vi "A-Lockin_Vsg.vi"(7 "Remote Lockin Address":string, 8 "error in (no error)":errorcluster, 11 "SweepControl.lvclass":refnum<class "SweepControl.lvclass">) -> (0 "error out":errorcluster)   [LabVIEW 2016, in "Transport.lvclass"]
uses:
  Transport.lvclass
  <userlib>/LevyLab/Lockin-Multichannel/Typedefs/AO-cluster.ctl
  <userlib>/LevyLab/Lockin-Multichannel/Typedefs/AO_Amp-array.ctl
  <userlib>/LevyLab/Lockin-Multichannel/Typedefs/AO_DC-array.ctl
  <userlib>/LevyLab/Lockin-Multichannel/Typedefs/AO_f-array.ctl
  <userlib>/LevyLab/Lockin-Multichannel/Typedefs/AO_phi-array.ctl
  <userlib>/LevyLab/Lockin-Multichannel/Typedefs/Function-array.ctl
  <userlib>/LevyLab/Lockin-Multichannel/Typedefs/Function-enum.ctl
  SweepControl/SweepControl.lvclass
  <userlib>/LevyLab/Levylab Instruments/Instrument Types/Cryostat/Instrument.Cryostat.lvclass
  <userlib>/LevyLab/LV to ITX/LVtoITX.lvclass
  Control Experiment/Control Experiment.lvclass
panel:
  in  "Tab Control":enum32{"lockin/SG Control", "Data", "Other"}(tab)
  out "elapsed time (s)":u32=76
  in  "Side Gate Channel(s)":i32[](array[numeric])
  in  "Channels: AO":T1={"AO amp (V)"=[0.0, 0.0, 0.0, 0.0, 0.0, 0.0, 0.0, 0.0], "AO DC (V)"=[0.0, 0.0, 0.0, 0.0, 0.0, 0.0, 0.0, 0.0], "AO f (Hz)"=[13.0, 13.0, 13.0, 13.0, 13.0, 13.0, 13.0, 13.0], "AO phi (°)"=[0.0, 0.0, 0.0, 0.0, 0.0, 0.0, 0.0, 0.0], "function"=[enum."Sine", enum."Sine", enum."Sine", enum."Sine", enum."Sine", enum."Sine", enum."Sine", enum."Sine"], "I+"=[]} {"AO f (Hz)" min=0.001 max=10000.0; "AO DC (V)" format="%.3p"; "AO amp (V)" format="%.3p"}
  in  "Vmax (end)":dbl=0.7 format="%#_3p"
  in  "Vmin (start)":dbl=-0.15 format="%#_3p"
  in  "dV":dbl=0.0005 format="%#_3p"
  in  "Experiment Comments":string="describe only the experiment you're doing right now"
  in  "Experiment folder":string="Experiment folder"
  out "T (mK)":dbl
  in  "wait after setting Vsg (ms)":u32
  in  "Initial wait (ms)":u32=10000
  in  "Physical Channel":tag="Dev2/ao0" caption="Back Gate Channel"
  in  "Sweep":enum16{"Vsg", "Vbg"}(ring)
  in  "cycles (1,2,...)":i32=1 min=1 step=1
  in  "phase":dbl
  out "ramp rate":dbl=0.2 format="%#_13g"
  out "Field (T)":dbl=0.5 format="%#_13g"
  in  "function (ramp)":enum16{"Ramp", "Triangle", "Sine"}(ring)
  in  "set \"Vsg\" to initial value?":bool
  out "time b/w points (ms)":u32=76
  in  "stop":bool
  out "X Lockins":cluster{"Y":dbl[], "Y":dbl[]}[](graph)
  in  "V1":i32=1 min=1
  in  "Current":i32=1 min=1
  in  "V2":i32=1 min=1
  out "X Lockins 2":cluster{"Y":dbl[], "Y":dbl[]}[](graph)
  out "G4T":cluster{"Y":dbl[], "Y":dbl[]}[](graph)
  # "1"
  # "2"
  # "3"
  # "4"
  # "5"
  # "6"
  # "7"
  # "8"
  # "If V1 /= V2:\nR = (V1-V2)/I\nIf V1 = V2:\nR = V1/I"
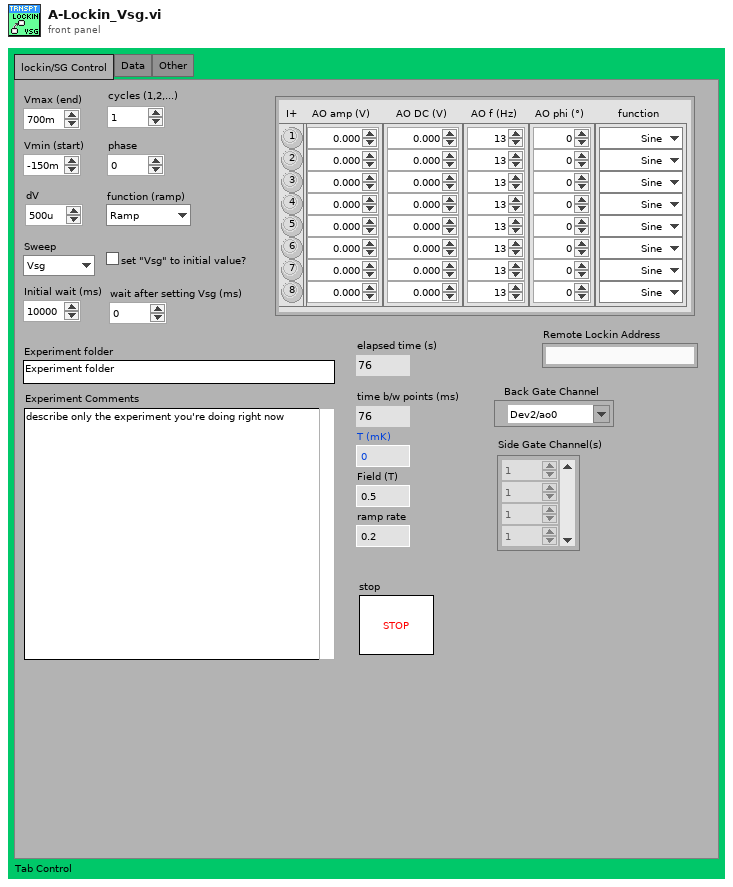
[diagram p1: front panel]
types:
  T1 = typedef "AO-cluster.ctl" = cluster{"AO amp (V)":T2, "AO DC (V)":T3, "AO f (Hz)":T4, "AO phi (°)":T5, "function":T6, "I+":bool[]}
  T2 = typedef "AO_Amp-array.ctl" = dbl[]
  T3 = typedef "AO_DC-array.ctl" = dbl[]
  T4 = typedef "AO_f-array.ctl" = dbl[]
  T5 = typedef "AO_phi-array.ctl" = dbl[]
  T6 = typedef "Function-array.ctl" = T7[]
  T7 = typedef "Function-enum.ctl" = enum16{"Sine", "Triangle", "Square", "Sawtooth"}
  T8 = cluster{"Temperature":refnum<class "Instrument.Cryostat.lvclass">, "Magnet":refnum<class "Instrument.Cryostat.lvclass">, "Rotator":refnum<class "Instrument.Cryostat.lvclass">, "Level":refnum<class "Instrument.Cryostat.lvclass">}
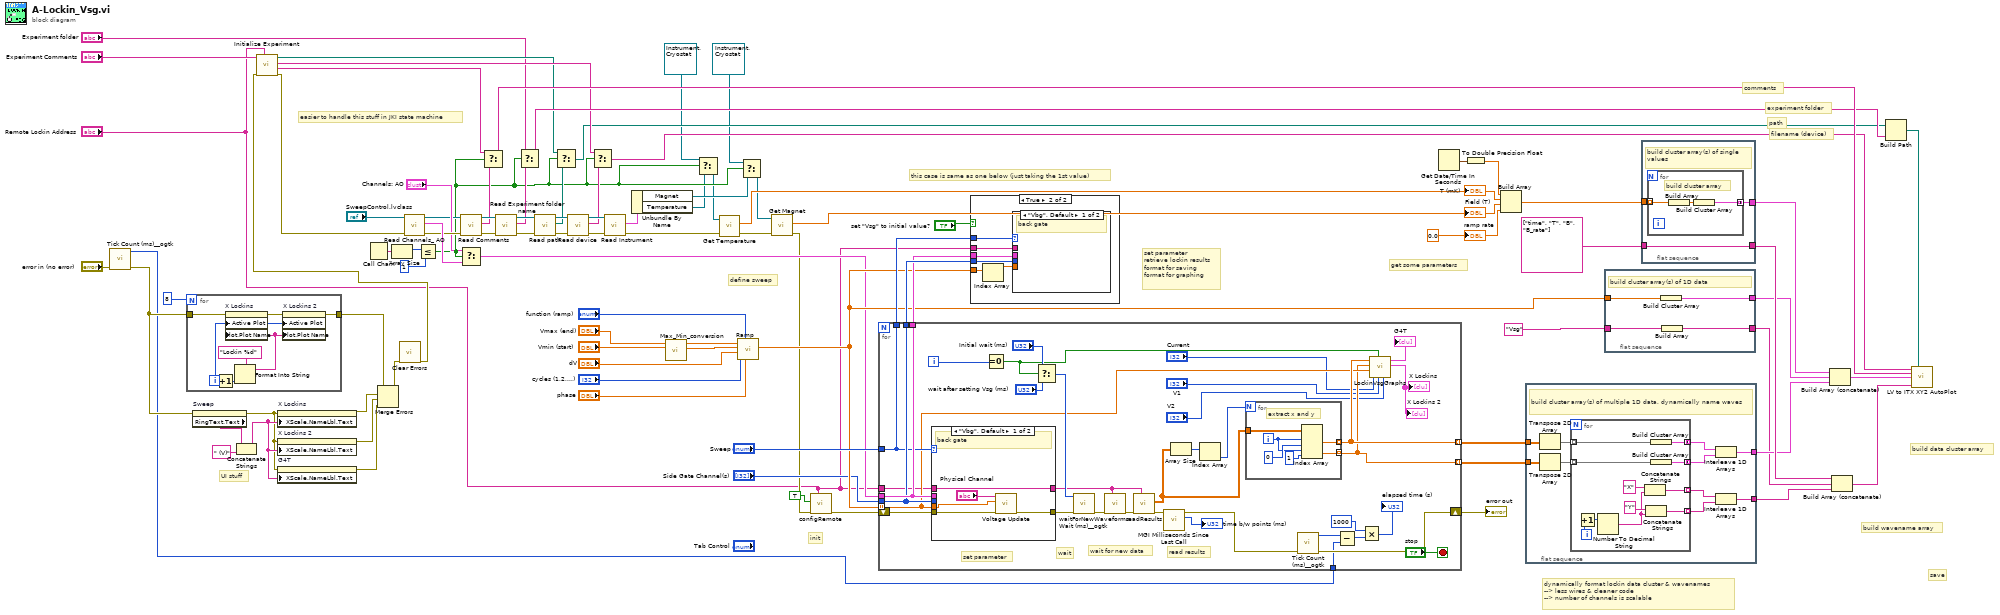
[diagram p0: block diagram]
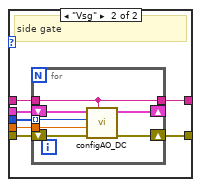
[diagram p2: hidden frame]
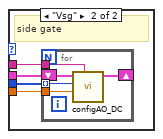
[diagram p4: hidden frame]
diagram:
  w69 = 0.0
  # "UI stuff"
  # "easier to handle this stuff in JKI state machine"
  # "filename (device)"
  # "path"
  # "comments"
  # "experiment folder"
  # "define sweep"
  # "get some parameters"
  # "set parameter\nretrieve lockin results\nformat for saving\nformat for graphing"
  # "save"
  # "this case is same as one below (just taking the 1st value)"
  # "init"
  # "build data cluster array"
  # "build wavename array"
  # "dynamically format lockin data cluster & wavenames\n--> less wires & cleaner code\n--> number of channels is scalable"
  n1 = call <userlib>:"Tick Count (ms)__ogtk.vi"("error in (no error)"="error in (no error)") -> ("error out"=w16:errorcluster, "millisecond timer value"=w4:u32)  [unwired: 9 in]
  n2 = for {
    N: 8 -> [_]
    tunnel: [w95] -> w10
    tunnel: w16 -> [w100]
    i -> [w98]
    n3 = Increment(x=w98) -> (x+1=w96:i32)
    n4 = Format Into String(format string="Lockin %d", w96) -> (resulting string=w99:string)  [unwired: 2 in, 1 out]
    n5 = property on="X Lockins" class="XYGraph (strict)"(error in=w100, "Active Plot"=w98, "Plot.Plot Name"=w99) -> (error out=w97:errorcluster)  [unwired: 1 in, 1 out]
    n6 = property on="X Lockins 2" class="XYGraph (strict)"(error in=w97, "Active Plot"=w98, "Plot.Plot Name"=w99) -> (error out=w95:errorcluster)  [unwired: 1 in, 1 out]
  }
  n7 = property on="Sweep" class="Enum (strict)"(error in=w16) -> (error out=w11:errorcluster, "RingText.Text"=w13:string)  [unwired: 1 in, 1 out]
  n8 = Concatenate Strings(w13, " (V)" ("string")) -> (w12:string)
  n9 = property on="X Lockins" class="XYGraph (strict)"(error in=w11, "XScale.NameLbl.Text"=w12) -> (error out=w9:errorcluster)  [unwired: 1 in, 1 out]
  n10 = property on="X Lockins 2" class="XYGraph (strict)"(error in=w11, "XScale.NameLbl.Text"=w12) -> (error out=w8:errorcluster)  [unwired: 1 in, 1 out]
  n11 = property on="G4T" class="XYGraph (strict)"(error in=w11, "XScale.NameLbl.Text"=w12) -> (error out=w7:errorcluster)  [unwired: 1 in, 1 out]
  n12 = Call Chain() -> (call chain=w64:string[])
  n13 = Merge Errors(w10, w9, w8, w7) -> (w6:errorcluster)
  n14 = Array Size(array=w64) -> (size(s)=w63:i32)
  n15 = call <vilib>:"Clear Errors.vi"("error in (no error)"=w6) -> ("error out"=w5:errorcluster)  [unwired: 5 in, 1 out]
  n16 = call "Initialize Experiment.vi"("lockin address"="Remote Lockin Address", "error in (no error)"=w5, "Experiment Comments"="Experiment Comments") -> ("error out"=w31:errorcluster, "Comments"=w32:string, "device"=w38:string, "path"=w36:path)  [unwired: 5 in]
  n17 = call-dynamic "Read Channels_ AO.vi"("error in (no error)"=w31, "SweepControl in"="SweepControl.lvclass") -> ("error out"=w56:errorcluster, "Channels: AO"=w61:T1, "SweepControl out"=w54:refnum<class "SweepControl.lvclass">)  [unwired: 7 in]
  n18 = Less Or Equal?(x=w63, y=1) -> (x <= y?=w23:bool)
  n19 = call-dynamic "Read Comments.vi"("error in (no error)"=w56, "SweepControl in"=w54) -> ("error out"=w58:errorcluster, "Comments"=w49:string, "SweepControl out"=w57:refnum<class "SweepControl.lvclass">)  [unwired: 7 in]
  n20 = Select(t="Channels: AO", s=w23, f=w61) -> (s? t:f=w59:T1)
  n21 = Select(t=w32, s=w23, f=w49) -> (s? t:f=w47:string)
  n22 = call-dynamic "Read Experiment folder name.vi"("error in (no error)"=w58, "SweepControl in"=w57) -> ("error out"=w53:errorcluster, "Experiment folder name"=w48:string, "SweepControl out"=w50:refnum<class "SweepControl.lvclass">)  [unwired: 7 in]
  n23 = Select(t="Experiment folder", s=w23, f=w48) -> (s? t:f=w41:string)
  n24 = call-dynamic "Read path.vi"("error in (no error)"=w53, "SweepControl in"=w50) -> ("error out"=w52:errorcluster, "path"=w40:path, "SweepControl out"=w51:refnum<class "SweepControl.lvclass">)  [unwired: 7 in]
  n25 = Select(t=w36, s=w23, f=w40) -> (s? t:f=w35:path)
  n26 = call-dynamic "Read device.vi"("error in (no error)"=w52, "SweepControl in"=w51) -> ("error out"=w45:errorcluster, "device"=w39:string, "SweepControl out"=w46:refnum<class "SweepControl.lvclass">)  [unwired: 7 in]
  n27 = Select(t=w38, s=w23, f=w39) -> (s? t:f=w37:string)
  n28 = call-dynamic "Read Instrument.vi"("error in (no error)"=w45, "SweepControl in"=w46) -> ("error out"=w28:errorcluster, "Instrument"=w24:T8)  [unwired: 7 in, 1 out]
  n29 = Unbundle By Name(w24) -> ("Magnet"=w22:refnum<class "Instrument.Cryostat.lvclass">, "Temperature"=w21:refnum<class "Instrument.Cryostat.lvclass">)
  n30 = call <userlib>:"Max_Min_conversion.vi"("Min"="Vmin (start)", "Max"="Vmax (end)") -> ("offset"=w91:dbl, "Amplitude"=w92:dbl)  [unwired: 8 in]
  n31 = Select(t=refnum<class "Instrument.Cryostat.lvclass"> refnum ("Magnet"), s=w23, f=w21) -> (s? t:f=w20:refnum<class "Instrument.Cryostat.lvclass">)
  n32 = call-dynamic "Get Temperature.vi"("error in (no error)"=w28, "Instrument.Cryostat in"=w20) -> ("error out"=w29:errorcluster, "Temperature (K)"=w25:dbl)  [unwired: 6 in, 2 out]
  "T (mK)" <- w25
  n33 = call <userlib>:"Ramp.vi"("phase"="phase", "function (ramp)"="function (ramp)", "cycles (1,2,...)"="cycles (1,2,...)", "step size"="dV", "offset"=w91, "amplitude"=w92) -> ("Waveform Graph"=w66:dbl[])  [unwired: 3 in, 2 out]
  n34 = Select(t=refnum<class "Instrument.Cryostat.lvclass"> refnum ("Magnet"), s=w23, f=w22) -> (s? t:f=w19:refnum<class "Instrument.Cryostat.lvclass">)
  n35 = call-dynamic "Get Magnet.vi"("error in (no error)"=w29, "Instrument.Cryostat in"=w19) -> ("error out"=w27:errorcluster, "B Field (T)"=w26:dbl)  [unwired: 6 in, 2 out]
  "Field (T)" <- w26
  n36 = call <userlib>:"configRemote.vi"("address"="Remote Lockin Address", "error in (no error)"=w27, "Remote Mode"=TRUE) -> ("error out"=w85:errorcluster)  [unwired: 8 in]
  n37 = for {
    tunnel: w59 -> [w136]
    tunnel: w66 -> [w119] mode=indexing
    tunnel: "Sweep" -> [w134]
    tunnel: "Side Gate Channel(s)" -> [w135]
    tunnel: [w136] -> w84
    tunnel: [w135] -> w87
    tunnel: [w134] -> w86
    shift-right: [w112] -> w80
    shift-left: w85 -> [w133]
    tunnel: [w121] -> w83 mode=indexing
    tunnel: [w118] -> w82 mode=indexing
    tunnel: w4 -> [w110]
    tunnel: "Remote Lockin Address" -> [w104]
    i -> [w131]
    stop <- "stop" stop-if-true
    # "read results"
    # "wait for new data"
    # "wait"
    # "set parameter"
    n38 = case shown="\"Vbg\", Default" w134 {
      tunnel: w136 -> [_ w148]
      tunnel: w119 -> [w137 w146]
      tunnel: w135 -> [_ w147]
      tunnel: w133 -> [w139 w145]
      tunnel: [w138 w144] -> w132
      tunnel: w104 -> [w141 w143]
      tunnel: [w141 w142] -> w103
      frame "Vbg", Default {
        # "back gate"
        n39 = call <vilib>:"Voltage Update.vi"("error in (no error)"=w139, "Voltage Output"=w137, "Physical Channel"="Physical Channel") -> ("error out"=w138:errorcluster)  [unwired: 7 in, 1 out]
      }
      frame "Vsg" {
        # "side gate"
        n40 = for {
          tunnel: w147 -> [w154] mode=indexing
          tunnel: w146 -> [w153]
          shift-right: [w151] -> w144
          shift-left: w145 -> [w152]
          shift-right: [w150] -> _
          shift-left: w148 -> [w155]
          tunnel: w143 -> [w149]
          tunnel: [w149] -> w142
          n41 = call <userlib>:"configAO_DC.vi"("address"=w149, "error in (no error)"=w152, "new DC (V)"=w153, "AO Channel"=w154, "Channels: AO"=w155) -> ("error out"=w151:errorcluster, "Channels: AO"=w150:T1)  [unwired: 5 in]
        }
      }
    }
    n42 = Equal To 0?(x=w131) -> (x = 0?=w120:bool)
    n43 = Select(t="Initial wait (ms)", s=w120, f="wait after setting Vsg (ms)") -> (s? t:f=w124:u32)
    n44 = call <userlib>:"Wait (ms)__ogtk.vi"("error in (no error)"=w132, "milliseconds to wait"=w124) -> ("error out"=w127:errorcluster)  [unwired: 8 in, 1 out]
    n45 = call <userlib>:"waitForNewWaveforms.vi"("address"=w103, "error in (no error)"=w127) -> ("error out"=w122:errorcluster)  [unwired: 8 in, 1 out]
    n46 = call <userlib>:"readResults.vi"("address"=w103, "error in (no error)"=w122) -> ("error out"=w130:errorcluster, "Results"=w102:dbl[][])  [unwired: 7 in, 1 out]
    n47 = call <userlib>:"MGI Milliseconds Since Last Call.vi"("Error In"=w130) -> ("ms"=→"time b/w points (ms)":u32, "Error Out"=w109:errorcluster)  [unwired: 5 in]
    n48 = Array Size(array=w102) -> (size(s)=w129:i32[])
    n49 = Index Array(array=w129) -> (element=w128:i32)  [unwired: 1 in]
    n50 = for {
      N: w128 -> [_]
      tunnel: w102 -> [w159]
      tunnel: [w157] -> w121 mode=indexing
      tunnel: [w156] -> w118 mode=indexing
      i -> [w158]
      # "extract x and y"
      n51 = Index Array(array=w159, index (row) #1=w158, index (col) #1=0 ("disabled index (col)"), index (row) #2=w158, index (col) #2=1 ("disabled index (col)")) -> (element #1=w157:dbl, element #2=w156:dbl)
    }
    n52 = call <userlib>:"Tick Count (ms)__ogtk.vi"("error in (no error)"=w109) -> ("error out"=w112:errorcluster, "millisecond timer value"=w111:u32)  [unwired: 9 in]
    n53 = Subtract(x=w111, y=w110) -> (x-y=w108:u32)
    n54 = Multiply(x=u32 1000, y=w108) -> (x*y=→"elapsed time (s)":u32)
    n55 = call "LockinVsgGraphs.vi"("V2"="V2", "V1"="V1", "reset?"=w120, "Current"="Current", "parameter in"=w119, "Y array in"=w118, "X array in"=w121) -> ("X vs Parameter"=→"X Lockins" →"X Lockins 2":cluster{"Y":dbl[], "Y":dbl[]}[], "G vs Parameter Out"=→"G4T":cluster{"Y":dbl[], "Y":dbl[]}[])  [unwired: 2 in, 1 out]
  }
  "error out" <- w80
  n56 = case shown="True" "set \"Vsg\" to initial value?" {
    tunnel: w84 -> [_ w167]
    tunnel: w66 -> [_ w166]
    tunnel: w87 -> [_ w164]
    tunnel: w86 -> [_ w165]
    tunnel: "Remote Lockin Address" -> [_ w162]
    frame False {
    }
    frame True {
      n57 = Index Array(array=w166) -> (element=w163:dbl)  [unwired: 1 in]
      n58 = case shown="\"Vbg\", Default" w165 {
        tunnel: w167 -> [_ w169]
        tunnel: w163 -> [_ w170]
        tunnel: w164 -> [_ w171]
        tunnel: w162 -> [_ w168]
        frame "Vbg", Default {
          # "back gate"
        }
        frame "Vsg" {
          # "side gate"
          n59 = for {
            tunnel: w171 -> [w176] mode=indexing
            tunnel: w170 -> [w175]
            shift-right: [w173] -> _
            shift-left: w169 -> [w174]
            tunnel: w168 -> [w172]
            n60 = call <userlib>:"configAO_DC.vi"("address"=w172, "new DC (V)"=w175, "AO Channel"=w176, "Channels: AO"=w174) -> ("Channels: AO"=w173:T1)  [unwired: 6 in, 1 out]
          }
        }
      }
    }
  }
  n61 = Get Date/Time In Seconds() -> (seconds since 1Jan1904=w72:timestamp)
  n62 = To Double Precision Float(number=w72) -> (double precision float=w70:dbl)
  n63 = Build Array(w70, w25, w26, w69) -> (w71:dbl[])
  n64 = flat-sequence {
    tunnel: w83 -> [w186]
    tunnel: w82 -> [w185]
    tunnel: [w178] -> w76
    tunnel: [w177] -> w75
    frame #0 {
      # "build cluster array(s) of multiple 1D data, dynamically name waves"
      n65 = Transpose 2D Array(2D array=w186) -> (transposed array=w184:dbl[][])
      n66 = Transpose 2D Array(2D array=w185) -> (transposed array=w183:dbl[][])
      n67 = for {
        tunnel: w184 -> [w197] mode=indexing
        tunnel: w183 -> [w196] mode=indexing
        tunnel: [w195] -> w182 mode=concatenating
        tunnel: [w194] -> w181 mode=concatenating
        tunnel: [w189] -> w180 mode=indexing
        tunnel: [w188] -> w179 mode=indexing
        i -> [w191]
        n68 = Increment(x=w191) -> (x+1=w187:i32)
        n69 = Number To Decimal String(number=w187) -> (decimal integer string=w190:string)  [unwired: 1 in]
        n70 = Concatenate Strings("X" ("wavenames"), w190) -> (w189:string)
        n71 = Concatenate Strings("Y" ("wavenames"), w190) -> (w188:string)
        n72 = Build Cluster Array(w197) -> (w195:cluster{dbl[]}[])
        n73 = Build Cluster Array(w196) -> (w194:cluster{dbl[]}[])
      }
      n74 = Interleave 1D Arrays(w182, w181) -> (w177:cluster{dbl[]}[])
      n75 = Interleave 1D Arrays(w180, w179) -> (w178:string[])
    }
  }
  n76 = flat-sequence {
    tunnel: [w198] -> w74
    tunnel: w66 -> [w201]
    tunnel: [w200] -> w73
    tunnel: "Vsg" ("wavenames") -> [w199]
    frame #0 {
      # "build cluster array(s) of 1D data"
      n77 = Build Cluster Array(w201) -> (w200:cluster{"Waveform Graph":dbl[]}[])
      n78 = Build Array(w199) -> (w198:string[])
    }
  }
  n79 = flat-sequence {
    tunnel: [w204] -> w79
    tunnel: [w202] -> w77
    tunnel: w71 -> [w203]
    tunnel: string[] ["time", "T", "B", "B_rate"] ("wavenames (.Vx, etc)") -> [w202]
    frame #0 {
      # "build cluster array(s) of single values"
      n80 = for {
        tunnel: [w206] -> w204 mode=concatenating
        tunnel: w203 -> [w205] mode=indexing
        # "build cluster array"
        n81 = Build Array(w205) -> (w207:dbl[])
        n82 = Build Cluster Array(w207) -> (w206:cluster{dbl[]}[])
      }
    }
  }
  n83 = Build Array (concatenate)(w79, w73, w75) -> (w78:cluster{"Waveform Graph":dbl[]}[])
  n84 = Build Array (concatenate)(w77, w74, w76) -> (w81:string[])
  n85 = Build Path(base path=w35, name or relative path=w41) -> (appended path=w94:path)
  n86 = call <userlib>:"LV to ITX XY2 AutoPlot.vi"("filename"=w37, "path"=w94, "Notes"=w47, "Data"=w78, "wavenames (.Vx, etc)"=w81) -> ()  [unwired: 10 in, 1 out]
  "ramp rate" <- w69
